vi "例3.6 下拉列表(简易计算器)2.vi"() -> ()   [LabVIEW 2017]
panel:
  in  "下拉列表":u16(ring) items=["相减", "相加", "相乘"]
  out "Result":dbl
  in  "B":dbl
  in  "A":dbl
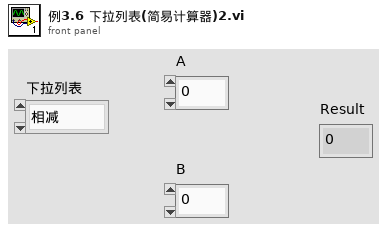
[diagram p1: front panel]
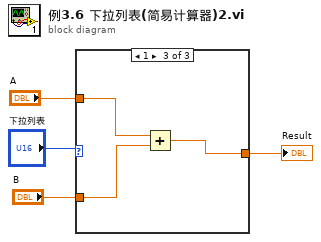
[diagram p0: block diagram]
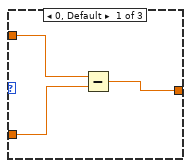
[diagram p2: hidden frame]
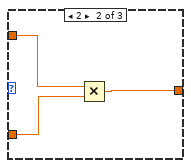
[diagram p3: hidden frame]
diagram:
  n1 = case shown="1" "下拉列表" {
    tunnel: "A" -> [w7 w10 w13]
    tunnel: "B" -> [w6 w9 w12]
    tunnel: [w5 w8 w11] -> w2
    frame 0, Default {
      n2 = Subtract(x=w7, y=w6) -> (x-y=w5:dbl)
    }
    frame 2 {
      n3 = Multiply(x=w10, y=w9) -> (x*y=w8:dbl)
    }
    frame 1 {
      n4 = Add(x=w13, y=w12) -> (x+y=w11:dbl)
    }
  }
  "Result" <- w2
